vi "Data Type to Persistence.vi"(8 "error in (no error)":errorcluster, 11 "Data Type":refnum<class "Data Type.lvclass">) -> (0 "error out":errorcluster, 3 "Persistence":refnum<class "IPersist.lvclass">)   [LabVIEW 2017, in "Custom Type Test Executive.lvlib" / "Persistence.lvclass"]
uses:
  <vilib>/gpm_packages/@cs/test-executive/Source/Custom Type Test Executive/Persistence Data Type/Persistence.lvclass
  <vilib>/gpm_packages/@cs/persistence/source/IPersist/IPersist.lvclass
  <vilib>/gpm_packages/@cs/data-type-serializer/source/Data Type/Data Type.lvclass
  <vilib>/gpm_packages/@cs/test-executive/Source/Custom Type Test Executive/Persistence Data Type/Persistence.lvclass/Persistence.ctl
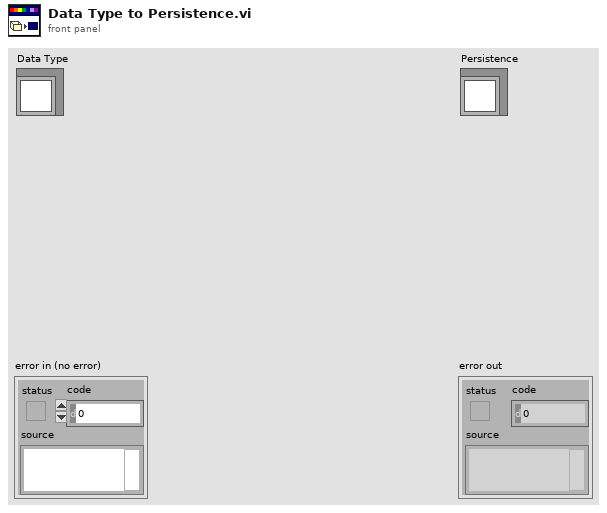
[diagram p1: front panel]
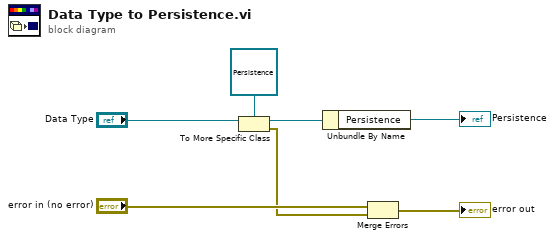
[diagram p0: block diagram]
diagram:
  n1 = To More Specific Class(target class=refnum<class "Persistence.lvclass"> refnum ("Boolean out"), reference="Data Type") -> (specific class reference=w4:refnum<class "Persistence.lvclass">, error out=w1:errorcluster)  [unwired: 1 in]
  n2 = Unbundle By Name(w4) -> ("Persistence"=→"Persistence":refnum<class "IPersist.lvclass">)
  n3 = Merge Errors("error in (no error)", w1) -> (→"error out":errorcluster)
